vi "Cmd Get Parameter Properties (CR).vi"(4 "error in (no error)":errorcluster, 6 "parameter index":variant, 7 "command-recordset reference":T4) -> (0 "error out":errorcluster, 1 "parameter properties":T1, 3 "command-recordset reference out":T4)   [LabVIEW 2012, in "NI_Database_API_64.lvlib"]
doc: "Gets properties of the object as determined by the inputs. This VI works for connections, commands, recordsets, columns, and parameters. Wire data to the reference input to determine the polymorphic instance to use or manually select the instance."
uses:
  NI_Database_API_64.lvlib
  Command-Recordset.llb/Cmd-Rec Object Reference.ctl
  Cmd Parameter Properties.ctl
  Auxilliary.llb/DB Tools DataTypes.ctl
  Auxilliary.llb/DB Tools Parameter Dir.ctl
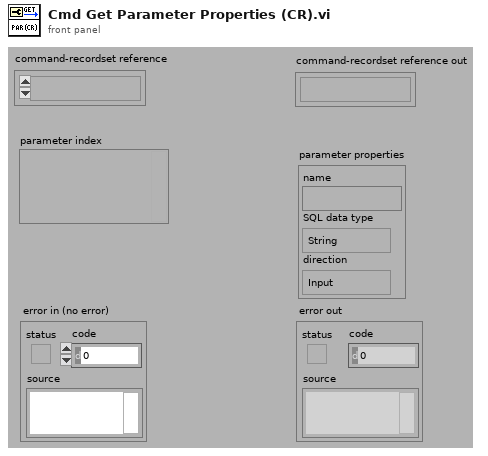
[diagram p1: front panel]
types:
  T1 = typedef "NI_Database_API_64.lvlib/Cmd Parameter Properties.ctl" = cluster{"name":string, "SQL data type":T2, "direction":T3}
  T2 = typedef "NI_Database_API_64.lvlib/DB Tools DataTypes.ctl" = enum16{"String", "Long (I32)", "Single (SGL)", "Double (DBL)", "Date/Time", "Binary"}
  T3 = typedef "NI_Database_API_64.lvlib/DB Tools Parameter Dir.ctl" = enum32{"Input", "Output", "Input/Output", "Return Value"}
  T4 = typedef "NI_Database_API_64.lvlib/Cmd-Rec Object Reference.ctl" = refnum<k1>
  T5 = typedef "NI_Database_API_64.lvlib/Cmd-Rec Data Members.ctl" = cluster{"recordset reference":T6, "command reference":T7}
  T6 = typedef "NI_Database_API_64.lvlib/Rec ObjectReference.ctl" = refnum<k1>
  T7 = typedef "NI_Database_API_64.lvlib/Cmd ObjectReference.ctl" = refnum<k1>
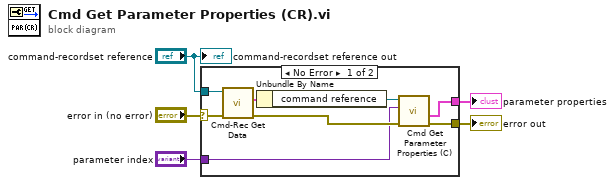
[diagram p0: block diagram]
diagram:
  n1 = case shown="No Error" "error in (no error)" {
    selector: "error in (no error)" -> [w6 w14]
    tunnel: [w13 w14] -> w5
    tunnel: [w12 _] -> w4
    tunnel: "command-recordset reference" -> [w8 _]
    tunnel: "parameter index" -> [w7 _]
    frame No Error {
      n2 = call "Cmd-Rec Get Data.vi"("error in (no error)"=w6, "command-recordset reference"=w8) -> ("error out"=w9:errorcluster, "data"=w10:T5)  [unwired: 2 in, 2 out]
      n3 = Unbundle By Name(w10) -> ("command reference"=w11:T7)
      n4 = call "Cmd Get Parameter Properties (C).vi"("error in (no error)"=w9, "parameter index"=w7, "command reference"=w11) -> ("error out"=w13:errorcluster, "parameter properties"=w12:T1)  [unwired: 2 in, 1 out]
    }
    frame Error {
    }
  }
  "error out" <- w5
  "parameter properties" <- w4
  "command-recordset reference out" <- "command-recordset reference"
